vi "getTestInfoFromDB.vi"(6 "error in (no error)":errorcluster, 10 "Equipo.lvclass":refnum<class "Equipo.lvclass">) -> (0 "error out":errorcluster, 1 "DescripcionPruebas":string[](array[string]), 2 "NombrePruebas":string[](array[string]), 3 "Base de Datos out":refnum<class "Base de Datos.lvclass">)   [LabVIEW 2019, in "Base de Datos.lvclass"]
uses:
  Base de Datos.lvclass
  Equipo/Equipo/Equipo.lvclass
  <vilib>/Utility/file.llb/Read Delimited Spreadsheet (string).vi
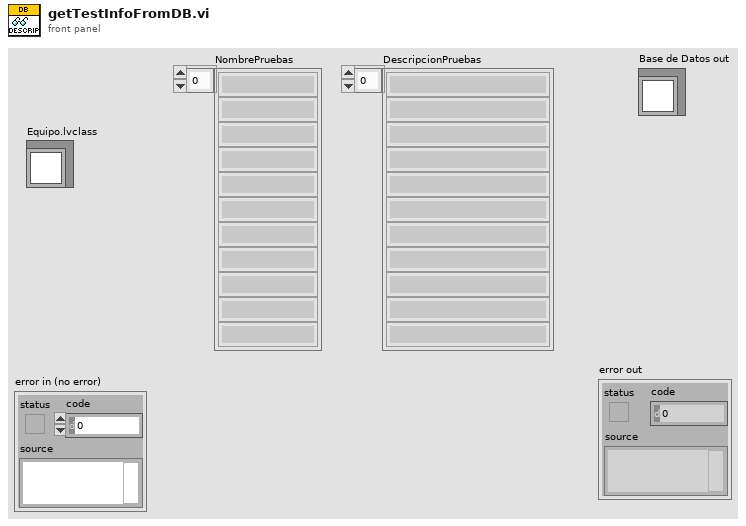
[diagram p1: front panel]
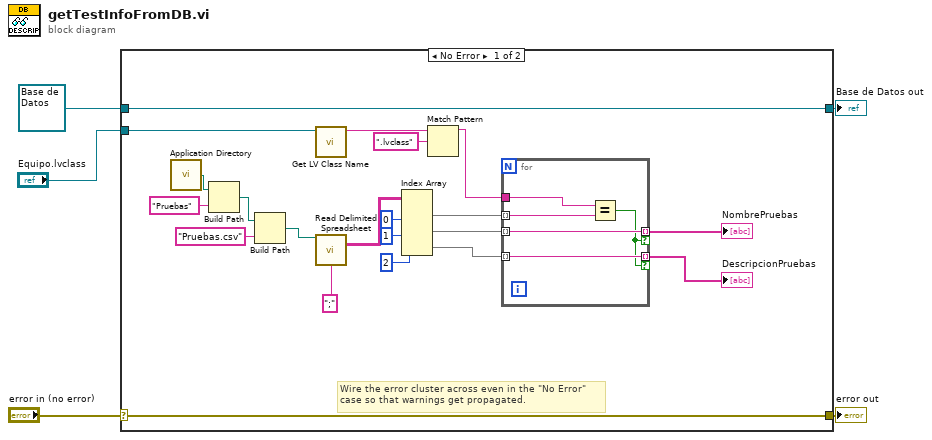
[diagram p0: block diagram]
diagram:
  n1 = case shown="No Error" "error in (no error)" {
    selector: "error in (no error)" -> [w25 w33]
    tunnel: [w25 w33] -> w4
    tunnel: [w26 w32] -> w2
    tunnel: refnum<class "Base de Datos.lvclass"> refnum ("Base de Datos in") -> [w26 w32]
    tunnel: "Equipo.lvclass" -> [w9 _]
    frame No Error {
      # "Wire the error cluster across even in the \"No Error\"\ncase so that warnings get propagated."
      n2 = call <vilib>:"Application Directory.vi"() -> ("Application Directory"=w24:path)
      n3 = Build Path(base path=w24, name or relative path="Pruebas") -> (appended path=w22:path)
      n4 = Build Path(base path=w22, name or relative path="Pruebas.csv") -> (appended path=w20:path)
      n5 = call <vilib>:"Get LV Class Name.vi"("object"=w9) -> ("class name"=w8:string)  [unwired: 9 in, 1 out]
      n6 = call-poly <vilib>:"Read Delimited Spreadsheet.vi"("file path (dialog if empty)"=w20, "delimiter (\\t)"=";" ("delimiter (\\t)")) -> ("all rows"=w18:string[][])  [unwired: 8 in, 5 out]
      n7 = Index Array(array=w18, index (col) #1=0 ("disabled index (col)"), index (col) #2=1 ("index (col)"), index (col) #3=2 ("index (col)")) -> (element #1=w14:string[], element #2=w13:string[], element #3=w12:string[])  [unwired: 3 in]
      n8 = Match Pattern(string=w8, regular expression=".lvclass") -> (before substring=w6:string)  [unwired: 1 in, 3 out]
      n9 = for {
        tunnel: w14 -> [w31] mode=indexing
        tunnel: [w30] -> w10 mode=indexing if=w28
        tunnel: w13 -> [w30] mode=indexing
        tunnel: w12 -> [w29] mode=indexing
        tunnel: [w29] -> w11 mode=indexing if=w28
        tunnel: w6 -> [w27]
        n10 = Equal?(x=w27, y=w31) -> (x = y?=w28:bool)
      }
      "NombrePruebas" <- w10
      "DescripcionPruebas" <- w11
    }
    frame Error {
    }
  }
  "error out" <- w4
  "Base de Datos out" <- w2
